vi "Create example IMAQ flattened string.vi"() -> (3 "U8StringImage":u8[](array[numeric]))   [LabVIEW 2020]
panel:
  out "size(s)":i32
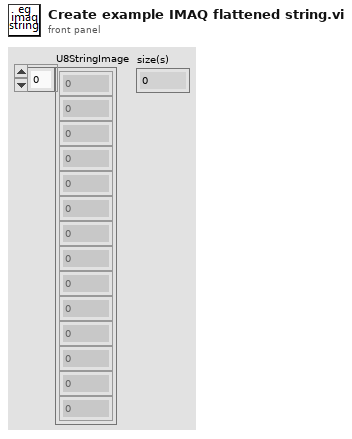
[diagram p1: front panel]
types:
  T1 = typedef "Image Type" = u32
  T2 = typedef "IMAQ Image.ctl" = refnum<image>
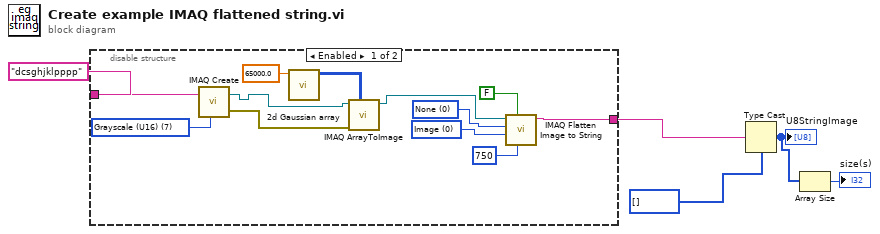
[diagram p0: block diagram]
diagram:
  n1 = disable-structure shown="Enabled" {
    disable-tunnel: "dcsghjklpppp" ("Image Name") -> [w11 w18]
    disable-tunnel: [w10 w18] -> w3
    frame Enabled {
      w12 = T1 7 items=["Grayscale (U8)", "Grayscale (I16)", "Grayscale (SGL)", "Complex (CSG)", "RGB (U32)", "HSL (U32)", "RGB (U64)", "Grayscale (U16)"] ("Image Type")
      w8 = 0 items=["None", "JPEG", "PACKED BINARY"] ("Compression (None)")
      w7 = 0 items=["Image", "Image and Vision Info", "Reference to Image"] ("Type of Flatten (Image and Vision Info)")
      n2 = call "IMAQ Create"("Image Name"=w11, "Image Type"=w12) -> ("New Image"=w15:T2, "error out"=w16:errorcluster)  [unwired: 3 in]
      n3 = call "2d Gaussian array.vi"("A"=65000.0) -> ("Intensity Graph"=w13:u16[][])  [unwired: 10 in]
      n4 = call "IMAQ ArrayToImage"("Image Pixels (U16)"=w13, "error in (no error)"=w16, "Image"=w15) -> ("Image Out"=w17:T2)  [unwired: 7 in, 1 out]
      n5 = call "IMAQ Flatten Image to String"("Quality (750)"=750, "Flatten with Process-Unique Name (F)"=FALSE, "Type of Flatten (Image and Vision Info)"=w7, "Compression (None)"=w8, "Image"=w17) -> ("Data String"=w10:string)  [unwired: 5 in, 1 out]
    }
    frame Disabled {
    }
  }
  n6 = Type Cast(type=u8[] [], x=w3) -> (*(type *) &x=w2:u8[])
  "U8StringImage" <- w2
  n7 = Array Size(array=w2) -> (size(s)=→"size(s)":i32)
